vi "Отредактируй меня.vi"() -> ()   [LabVIEW 2017]
doc: "This VI is part of Execise 10-3 of the LabVIEW Basics I course.\n\nThis VI is designed to help LabVIEW users discover creative ways of getting out of the jams they can get themselves into. If you can Edit this VI, you'll be able to access almost any VI, no matter how many features have been disabled in the VI Setup. Good Luck!"
panel:
  out "Display":string
  in  "Boolean":bool
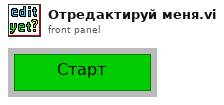
[diagram p1: front panel]
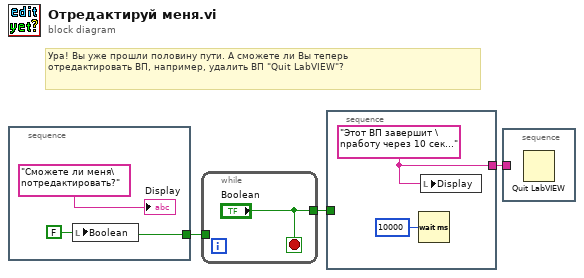
[diagram p0: block diagram]
diagram:
  # "Ура! Вы уже прошли половину пути. А сможете ли Вы теперь \nотредактировать ВП, например, удалить ВП \"Quit LabVIEW\"?"
  n1 = stacked-sequence {
    tunnel: [w4] -> w3
    frame #0 {
      w4 = FALSE ("Start")
      n2 = local write "Boolean"(w4) -> ()
      "Display" <- "Сможете ли меня\nотредактировать?"
    }
  }
  n3 = while {
    tunnel: ["Boolean"] -> w1
    tunnel: w3 -> [_]
    stop <- "Boolean" stop-if-true
  }
  n4 = stacked-sequence {
    tunnel: [w8] -> w2
    tunnel: w1 -> [_]
    frame #0 {
      w8 = "Этот ВП завершит \nработу через 10 сек..."
      n5 = Wait (ms)(milliseconds to wait=u32 10000) -> ()  [unwired: 1 out]
      n6 = local write "Display"(w8) -> ()
    }
  }
  n7 = stacked-sequence {
    tunnel: w2 -> [_]
    frame #0 {
      n8 = Quit LabVIEW() -> ()  [unwired: 1 in]
    }
  }
